vi "Stimulus-Create (full array).vi"(0 "StimChan":T1[](xcontrol), 1 "Apply multipliers? (F)":bool, 5 "Sampling Rate (Hz)":dbl=100000.0, 7 "Npts":i32=500, 9 "Rep Num":i32=-1, 11 "error in (no error)":errorcluster, 12 "Zero unused (F)":bool) -> (4 "StimChan Out":T1[](xcontrol), 6 "Waveform":dbl[][](array[numeric]), 8 "Multipliers":dbl[](array[numeric]), 15 "error out":errorcluster)   [LabVIEW 2020]
uses:
  Controls/Multichannel (Full)/Multichannel (Full).xctl
  Controls/Waveform XCtl/Waveform Enum.ctl
  PXI DAQ VIs/DAQ Engine VIs/AO Gain and Multiplier VIs/PXI Multipliers to AO Gains (1D).vi
panel:
  out "Ceilings":dbl[](array[numeric])
  out "Gains":dbl[](array[numeric])
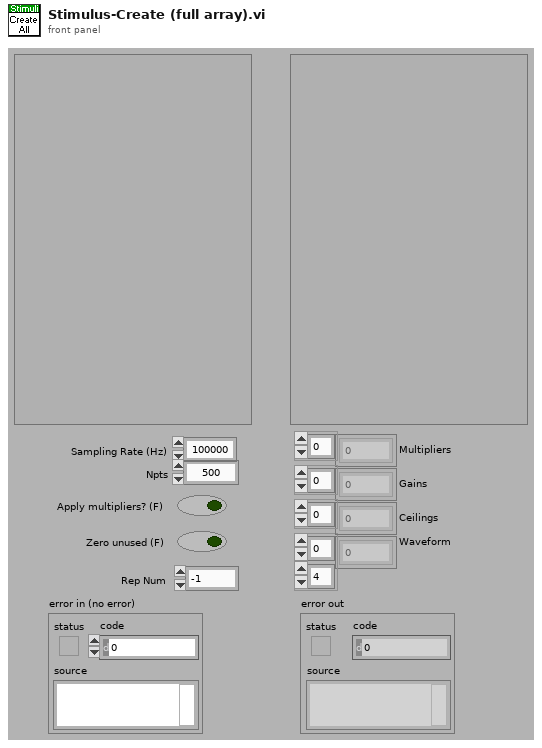
[diagram p1: front panel]
types:
  T1 = typedef "Stimulus Channel (Full).xctl/Full Stimulus Channel Data.ctl" = cluster{"Waveform":T2, "Filter":T19, "Burst":T21, "Level":T22, "Name":string, "Advanced":T24, "SAM":T25}
  T2 = typedef "Waveform XCtl.xctl/Waveform Data.ctl" = cluster{"Type":T3, "Tone":T4, "Pulse Train":T5, "Noise":T8, "File":T9, "FMSweep":T10, "Chirp Train":T11, "Complex Tone":cluster{"Params":T13, "Data":T15}, "Moving Ripple":T16}
  T3 = typedef "Waveform Enum.ctl" = enum16{"OFF", "Tone", "Noise", "Pulse Train", "File", "FM Sweep", "Chirp Train", "Complex Tone", "FM Tone", "Moving Ripple"}
  T4 = typedef "Tone Params.ctl" = cluster{"Frequency (kHz)":dbl, "Last Freq":dbl, "Last Phase":dbl}
  T5 = typedef "Pulse Train Params.ctl" = cluster{"Pulse width (us)":dbl, "Pulse rate (Hz)":dbl, "Gap (ms)":dbl, "Polarity":T6, "PT State":T7, "Asynch":bool}
  T6 = typedef "Pulse Polarity.ctl" = enum16{"POS", "NEG", "POS-NEG", "NEG-POS"}
  T7 = typedef "PT-Continuous State.ctl" = cluster{"Template":dbl[], "Nperiod":i32, "Index":i32, "Pulse Rate (Hz)":dbl, "Phase (cycles)":dbl, "Noff":i32}
  T8 = typedef "Noise Params.ctl" = cluster{"InvFilt":bool, "Noise":dbl[], "CurPt":i32, "Aweight":bool, "Seed":i32, "afile":path}
  T9 = typedef "StimFile-Params.ctl" = cluster{"Filename":path, "Signal":dbl[], "Channel":i32, "stream":bool, "offset":i32, "nreps":i32, "loops":i32, "Randomize":bool, "order":i32[], "Seed":i32, "Tokens":i32}
  T10 = typedef "FM Sweep Params.ctl" = cluster{"Rate (oct/s)":dbl, "Fmin (Hz)":dbl, "Fmax (Hz)":dbl, "Ramp (ms)":dbl, "Linear":bool}
  T11 = typedef "Chirp Train.ctl" = cluster{"Params":T12, "Data":cluster{"WF":dbl[]}}
  T12 = typedef "Chirp Train Params.ctl" = cluster{"Fmin (kHz)":dbl, "Fmax (kHz)":dbl, "Compensate":bool, "Duration (ms)":dbl}
  T13 = typedef "CT-Params.ctl" = cluster{"F0 (Hz)":dbl, "Band":cluster{"Flow (Hz)":dbl, "Fhigh (Hz)":dbl}, "Phase":T14, "Min F0 (Hz)":dbl, "Max F0 (Hz)":dbl, "ContinRandPhase":bool, "Max peak factor":dbl, "Max mod depth":dbl, "MinHarmNum":i32, "MaxHarmNum":i32, "Level Mode":enum16{"per component", "overall rms"}, "% jitter":dbl}
  T14 = typedef "CT-Phase Enum.ctl" = enum16{"Cosine", "Random", "Alternating"}
  T15 = typedef "CT-Runtime Data.ctl" = cluster{"Ncomp":i32, "MinHarm":i32, "Phase":dbl[], "Amplitude":dbl[], "Npts/frame":i32, "Last F0":dbl, "Fmin":dbl, "Fmax":dbl, "Lslope":dbl, "randphase":bool, "overall rms":bool, "fmult":dbl[], "jittered":bool}
  T16 = typedef "Moving Ripple.ctl" = cluster{"Params":T17, "Data":T18}
  T17 = typedef "Moving Ripple.Params.ctl" = cluster{"Fmin":dbl, "Fmax":dbl, "Density":dbl, "Velocity":dbl, "Depth":dbl, "Phase":dbl, "Comp/oct":i32}
  T18 = typedef "Moving Ripple.Data.ctl" = cluster{"Freq":dbl[], "A":dbl[], "phase":dbl[], "Phase":dbl}
  T19 = typedef "Advanced Filter XCtl.xctl/Filter Data.ctl" = cluster{"Type":enum16{"Lowpass", "Highpass", "Bandpass", "Bandstop", "OFF"}, "CF (kHz)":dbl, "BW (kHz)":dbl, "Cascade":bool, "Quadrature":bool, "Scale Factor":dbl, "Stages":cluster{"IIR Filter":cluster{"filter structure":enum32{"IIR 2nd Order", "IIR 4th Order"}, "Reverse Coefficients":dbl[], "Forward Coefficients":dbl[]}, "State":dbl[]}[], "Class":enum16{"Elliptic", "Butterworth"}, "Order":i32, "BWUnits":T20}
  T20 = typedef "Filter-Bandwidth Units.ctl" = enum16{"Linear", "Octaves", "Min-Max"}
  T21 = typedef "Burst Control.xctl/Burst Data.ctl" = cluster{"Active":bool, "Delay (ms)":dbl, "Duration (ms)":dbl, "Ramp (ms)":dbl, "Rate (Hz)":dbl, "Trepeat (ms)":dbl, "Repeat":bool}
  T22 = typedef "Level XCtl.xctl/Level Data.ctl" = cluster{"Level":dbl, "Units":T23, "Max":dbl, "Multiplier":dbl, "Cal File":path, "Cal":cluster{"Freq (Hz)":dbl[], "Mag (dB SPL)":dbl[], "Phase (deg)":dbl[]}}
  T23 = typedef "Level Units.ctl" = enum16{"dB atten", "dB SPL", "dB re 1 Vrms", "dB V/Hz½", "mW", "dB HL", "Volts", "dB mW"}
  T24 = typedef "Advanced Stimulus Options.xctl/Advanced Stimulus Options.ctl" = cluster{"Rep Mask":string, "AltPol":bool, "Var":string, "Expr":string, "Persist":bool}
  T25 = typedef "SAM Params.ctl" = cluster{"Active":bool, "Frequency (Hz)":dbl, "Depth":dbl, "Init Phase (cycles)":dbl, "phase (degrees)":dbl, "Asynch":bool}
  T26 = cluster{"Waveform":T2, "Filter":T19, "Burst":T21, "Level":T22, "Name":string, "Advanced":T24, "SAM":T25}
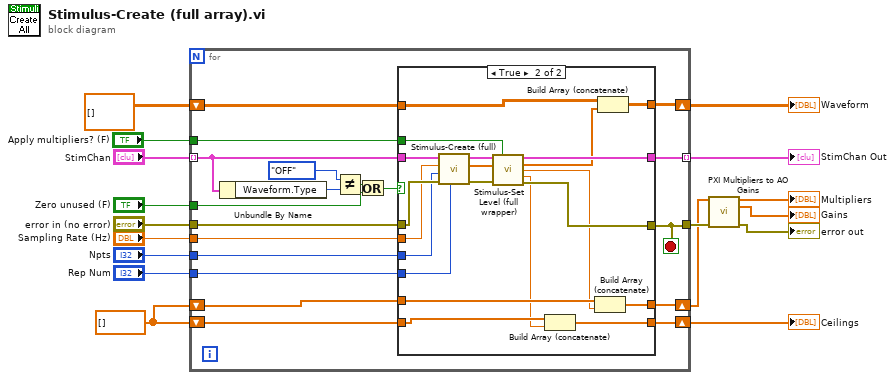
[diagram p0: block diagram]
diagram:
  w13 = dbl[] []
  n1 = for {
    tunnel: [w35] -> w3 mode=indexing
    shift-right: [w33] -> w6
    shift-left: dbl[][] [] ("Waveform") -> [w34]
    shift-right: [w31] -> w1
    shift-left: w13 -> [w32]
    shift-right: [w29] -> w12
    shift-left: w13 -> [w30]
    tunnel: "StimChan" -> [w28] mode=indexing
    tunnel: "Sampling Rate (Hz)" -> [w27]
    tunnel: "Npts" -> [w26]
    tunnel: "Zero unused (F)" -> [w21]
    tunnel: "Apply multipliers? (F)" -> [w20]
    tunnel: "error in (no error)" -> [w36]
    tunnel: [w19] -> w2
    tunnel: "Rep Num" -> [w18]
    stop <- w19 stop-if-true
    n2 = Unbundle By Name(w28) -> ("Waveform.Type"=w25:T3)
    n3 = Not Equal?(x=Waveform_Enum."OFF", y=w25) -> (x != y?=w24:bool)
    n4 = Or(x=w24, y=w21) -> (x .or. y?=w22:bool)
    n5 = case shown="True" w22 {
      tunnel: w36 -> [w40 w61]
      tunnel: [w40 w52] -> w19
      tunnel: [w37 w51] -> w35
      tunnel: w34 -> [w41 w59]
      tunnel: [w41 w60] -> w33
      tunnel: w32 -> [w39 w57]
      tunnel: [w39 w58] -> w31
      tunnel: w30 -> [w38 w55]
      tunnel: [w38 w56] -> w29
      tunnel: w28 -> [w37 w44]
      tunnel: w27 -> [_ w53]
      tunnel: w26 -> [_ w54]
      tunnel: w20 -> [_ w43]
      tunnel: w18 -> [_ w42]
      frame False {
      }
      frame True {
        n6 = call "Stimulus-Create (full).vi"("Rep Num"=w42, "error in (no error)"=w61, "Npts"=w54, "Sampling Rate (Hz)"=w53, "Stimulus Channel"=w44) -> ("error out"=w49:errorcluster, "Waveform"=w48:dbl[], "Stimulus Channel out"=w50:T26)  [unwired: 3 in, 1 out]
        n7 = call "Stimulus-Set Level (full wrapper).vi"("Stimulus Channel"=w50, "Apply multiplier? (F)"=w43, "Waveform in"=w48, "error in (no error)"=w49) -> ("Stimulus Channel out"=w51:T26, "Waveform out"=w45:dbl[], "Multiplier"=w46:dbl, "Ceiling"=w47:dbl, "error out"=w52:errorcluster)  [unwired: 7 in]
        n8 = Build Array (concatenate)(w55, w47) -> (w56:dbl[])
        n9 = Build Array (concatenate)(w57, w46) -> (w58:dbl[])
        n10 = Build Array (concatenate)(w59, w45) -> (w60:dbl[][])
      }
    }
  }
  "Waveform" <- w6
  "StimChan Out" <- w3
  "Ceilings" <- w12
  n11 = call-poly "PXI Multipliers to AO Gains.vi"("Multipliers in"=w1, "error in (no error)"=w2) -> ("Multipliers out"=→"Multipliers":dbl[], "Gains"=→"Gains":dbl[], "error out"=→"error out":errorcluster)  [unwired: 11 in]
